vi "Modified Framework AddNode.vi"(7 "parameters":variant, 8 "error in":errorcluster, 9 "node in":refnum<class "NISE_CEF_Node.lvclass">, 10 "parent node ID":string) -> (0 "error out":errorcluster, 2 "summary":T1[](array[typedef]), 3 "ID of Added Node":string)   [LabVIEW 2015, in "Configuration Tool.lvlib"]
doc: "This Vi adds a new node to the Parent Node IDCopyright 2015 National Instruments Corporation\n\nLicensed under the Apache License, Version 2.0 (the \"License\"); you may not use this file except in compliance with the License. You may obtain a copy of the License at http://www.apache.org/licenses/LICENSE-2.0\nUnless required by applicable law or agreed to in writing, software distributed under the License is distributed on an \"AS IS\" BASIS, WITHOUT WARRANTIES OR CONDITIONS OF ANY KIND, either express or implied. See the License for the specific language governing permissions and limitations under the License."
uses:
  Configuration Tool.lvlib
  <vilib>/NI/Configuration Framework/Node/Summary.ctl
  <vilib>/NI/Configuration Framework/Node/NISE_CEF_Node.lvclass
  <vilib>/NI/Configuration Framework/Node/NISE_CEF_Node.lvclass/NISE_CEF_Node.ctl
  <vilib>/NI/Configuration Framework/Node/ReadChildren.vi
  <vilib>/NI/Configuration Framework/Node/WriteParent.vi
  <vilib>/NI/Configuration Framework/NISE_CEF_TreeControl.lvlib
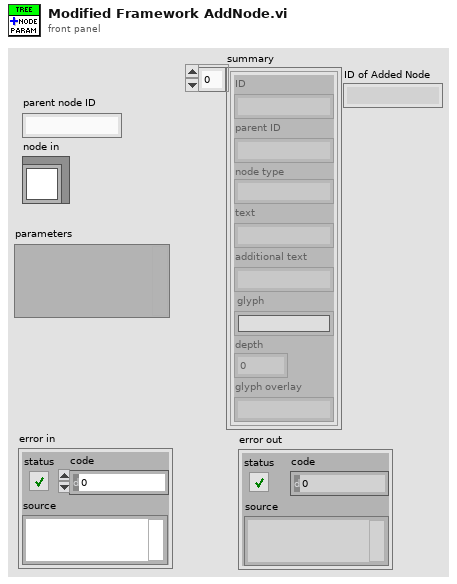
[diagram p1: front panel]
types:
  T1 = typedef "NISE_CEF_Node.lvclass/Summary.ctl" = cluster{"ID":string, "parent ID":string, "node type":string, "text":string, "additional text":string, "glyph":string, "depth":i32, "glyph overlay":string}
  T2 = typedef "NISE_CEF_Node.lvclass/NodeRef.ctl" = refnum<data-value>
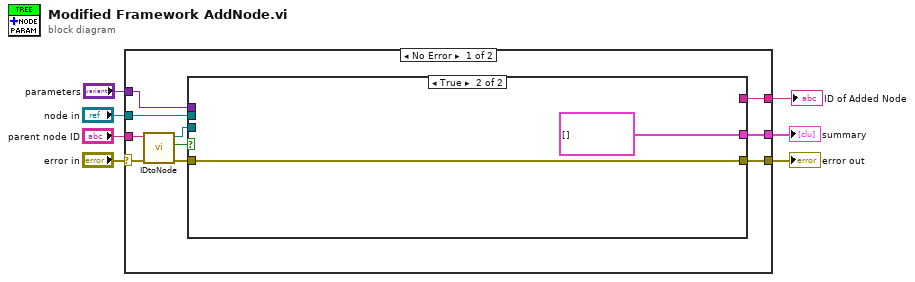
[diagram p0: block diagram]
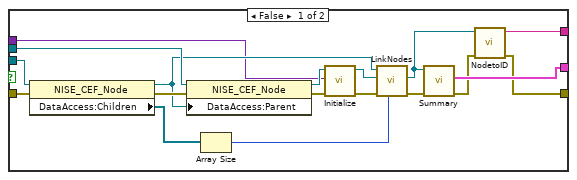
[diagram p2: hidden frame]
diagram:
  n1 = case shown="No Error" "error in" {
    selector: "error in" -> [w12 w38]
    tunnel: "parent node ID" -> [w17 _]
    tunnel: [w15 _] -> w5
    tunnel: [w14 w38] -> w4
    tunnel: "node in" -> [w13 _]
    tunnel: "parameters" -> [w9 _]
    tunnel: [w8 _] -> w1
    frame No Error {
      n2 = call <vilib>:"IDtoNode.vi"("error in"=w12, "ID"=w17) -> ("error out"=w11:errorcluster, "invalid Id"=w10:bool, "node ref"=w16:T2)  [unwired: 7 in]
      n3 = case shown="True" w10 {
        tunnel: w16 -> [w31 _]
        tunnel: [w35 T1[] [] ("summary")] -> w15
        tunnel: [w19 w37] -> w14
        tunnel: w13 -> [w25 _]
        tunnel: w11 -> [w28 w37]
        tunnel: w9 -> [w22 _]
        tunnel: [w18 _] -> w8
        frame False {
          n4 = property class="NISE_CEF_Node"(reference=w31, error in=w28) -> (reference out=w23:T2, error out=w27:errorcluster, "DataAccess:Children"=w30:T2[])
          n5 = property class="NISE_CEF_Node"(reference=w25, error in=w27, "DataAccess:Parent"=w23) -> (reference out=w24:refnum<class "NISE_CEF_Node.lvclass">, error out=w26:errorcluster)
          n6 = Array Size(array=w30) -> (size(s)=w29:i32)
          n7 = call-dynamic "Initialize.vi"("error in"=w26, "parameters"=w22, "node in"=w24) -> ("error out"=w32:errorcluster, "data value reference"=w33:T2)  [unwired: 6 in, 1 out]
          n8 = call <vilib>:"LinkNodes.vi"("index"=w29, "error in"=w32, "child in"=w33, "parent in"=w23) -> ("error out"=w34:errorcluster, "child out"=w21:T2)  [unwired: 5 in, 1 out]
          n9 = call <vilib>:"Summary.vi"("error in"=w34, "node self ref"=w21) -> ("error out"=w20:errorcluster, "summary"=w35:T1[])  [unwired: 8 in]
          n10 = call <vilib>:"NodetoID.vi"("error in"=w20, "node ref"=w21) -> ("error out"=w19:errorcluster, "ID"=w18:string)  [unwired: 8 in]
        }
        frame True {
        }
      }
    }
    frame Error {
    }
  }
  "error out" <- w4
  "summary" <- w5
  "ID of Added Node" <- w1
